vi "DWF PS Close.vi"(0 "Instrument Handle In":u32, 11 "Error In":errorcluster caption="Error In (no error)") -> (15 "Error Out":errorcluster)   [LabVIEW 2015, in "DigilentWF.lvlib"]
doc: "Stops the session and deallocates any resources acquired during the session. If output is enabled on any channels, they remain in their current state and continue to output data."
uses:
  <vilib>/DigilentWF/DigilentWF.lvlib
  dwf.dll
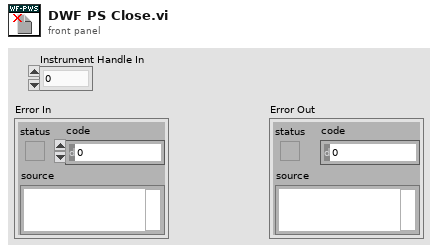
[diagram p1: front panel]
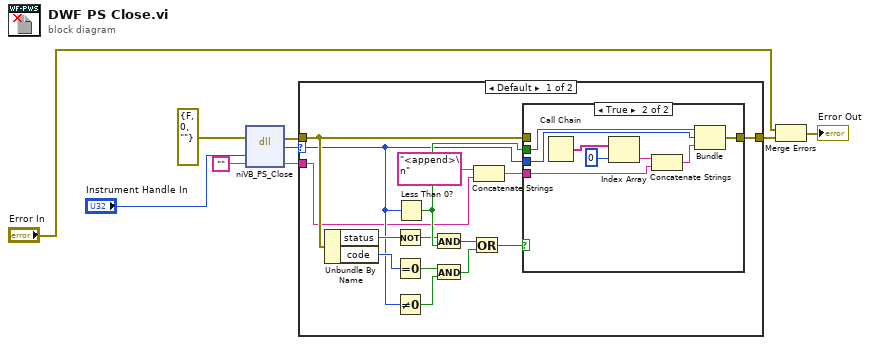
[diagram p0: block diagram]
diagram:
  n1 = dll-call lib="dwf.*" fn="niVB_PS_Close"(error in=errorcluster {"status"=FALSE, "code"=0, "source"=""} ("error in (no error)"), "instrumentHandleIn"="Instrument Handle In", "szError"="") -> (error out=w5:errorcluster, "return type"=w3:i32, "szError"=w2:string)  [unwired: 3 in, 1 out]
  n2 = case "inner_case" shown="Default" w3 {
    selector: w3 -> [w14 _]
    tunnel: w5 -> [w15 w34]
    tunnel: [w11 w34] -> w8
    tunnel: w2 -> [w10 _]
    frame Default {
      n3 = Unbundle By Name(w15) -> ("status"=w19:bool, "code"=w23:i32)
      n4 = Not(x=w19) -> (.not. x?=w22:bool)
      n5 = Equal To 0?(x=w23) -> (x = 0?=w18:bool)
      n6 = Not Equal To 0?(x=w14) -> (x != 0?=w21:bool)
      n7 = Less Than 0?(x=w14) -> (x < 0?=w24:bool)
      n8 = And(x=w22, y=w24) -> (x .and. y?=w20:bool)
      n9 = And(x=w18, y=w21) -> (x .and. y?=w17:bool)
      n10 = Or(x=w20, y=w17) -> (x .or. y?=w16:bool)
      n11 = Concatenate Strings("<append>\n" ("string"), w10) -> (w13:string)
      n12 = case shown="True" w16 {
        tunnel: [w25 w32] -> w11
        tunnel: w14 -> [_ w31]
        tunnel: w24 -> [_ w30]
        tunnel: w15 -> [w25 _]
        tunnel: w13 -> [_ w26]
        frame False {
        }
        frame True {
          n13 = Call Chain() -> (call chain=w29:string[])
          n14 = Index Array(array=w29, index=0) -> (element=w28:string)
          n15 = Concatenate Strings(w28, w26) -> (w33:string)
          n16 = Bundle(w30, "return type"=w31, w33) -> (w32:cluster{bool, "return type":i32, string})  [unwired: 1 out]
        }
      }
    }
    frame 0 {
    }
  }
  n17 = Merge Errors("Error In", w8) -> (→"Error Out":errorcluster)
